vi "FPGAPowerMeasurementWriteDirectlyToFile.vi"() -> ()   [LabVIEW 2009]
panel:
  out "Voltage at FPGA":dynamicdata(graph)
  in  "Number of Waveforms to Average":i32
  in  "rate":dbl=2000000.0
  in  "number of samples":i32=2000000
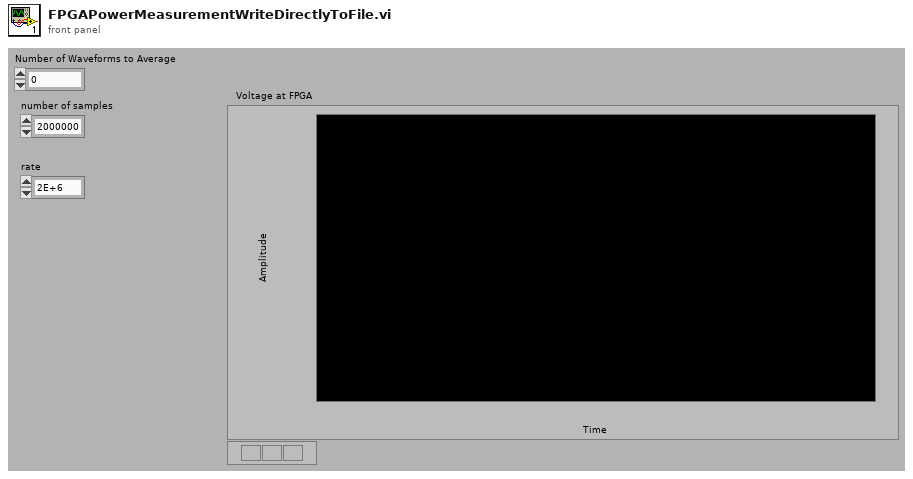
[diagram p1: front panel]
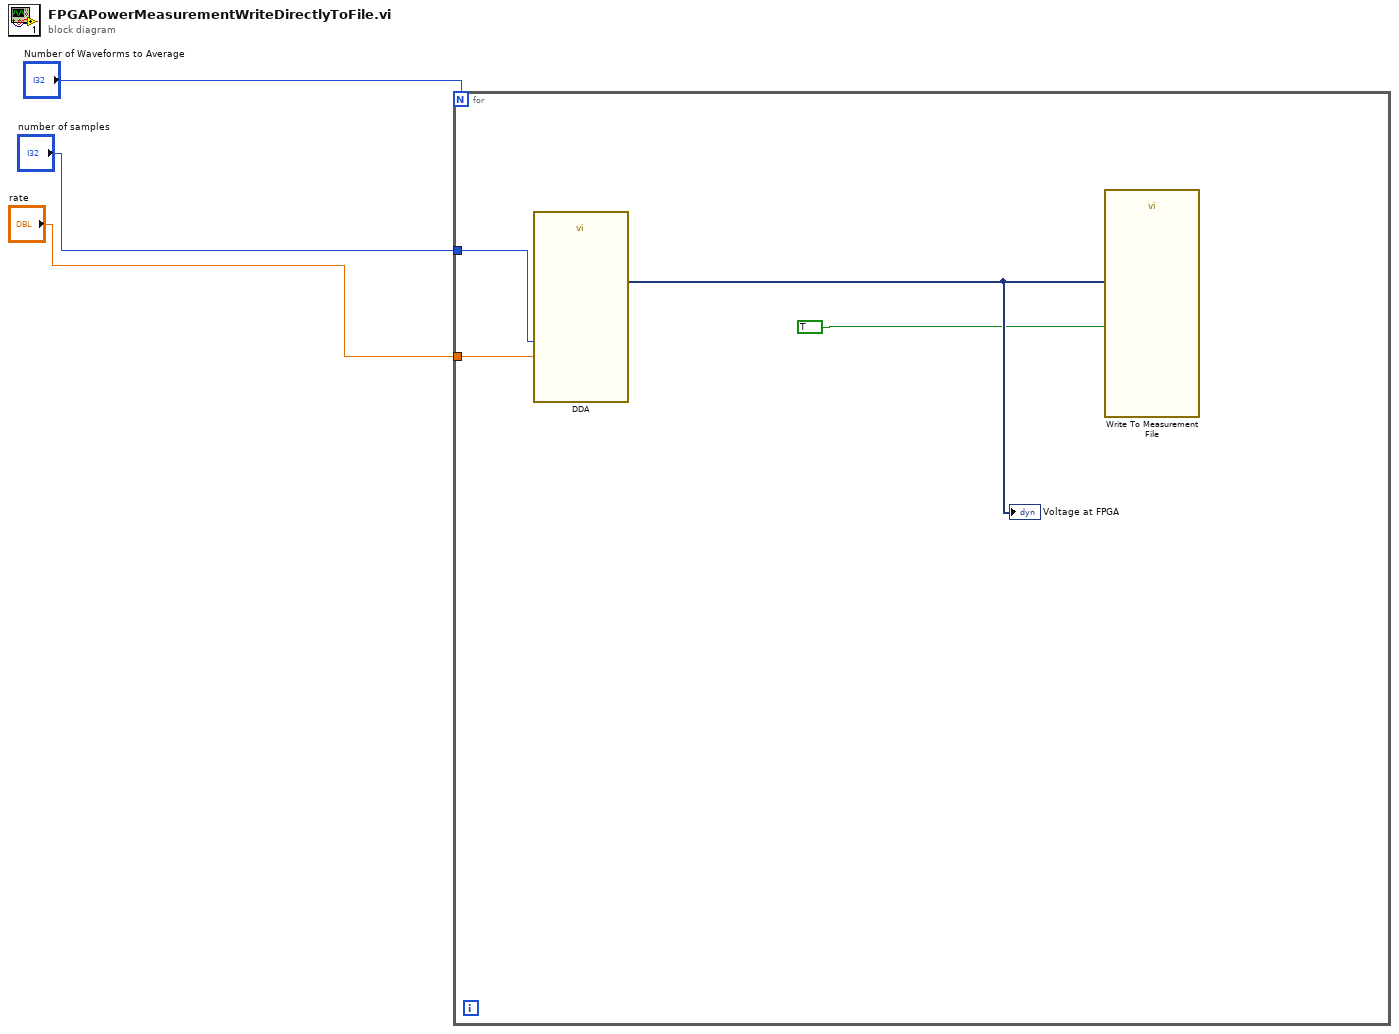
[diagram p0: block diagram]
diagram:
  n1 = for {
    N: "Number of Waveforms to Average" -> [_]
    tunnel: "number of samples" -> [w7]
    tunnel: "rate" -> [w6]
    n2 = call "DDA.vi"("rate"=w6, "number of samples"=w7) -> ("data"=w5:dynamicdata)  [unwired: 15 in, 2 out]
    "Voltage at FPGA" <- w5
    n3 = call "Write To Measurement File"("Signals"=w5, "Enable"=TRUE) -> ()  [unwired: 15 in, 3 out]
  }
